vi "TaskCreationEvents.vi"(8 "error in (no error)":errorcluster, 11 "DAQmx(AI) in":refnum<class "DAQmx(AI).lvclass">) -> (0 "error out":errorcluster, 3 "DAQmx(AI) out":refnum<class "DAQmx(AI).lvclass">)   [LabVIEW 2019, in "DAQmx(AI).lvclass"]
uses:
  DAQmx(AI).lvclass
  Typedefs/ScalingEvent--Cluster.ctl
  Typedefs/Scaling(MapRange)--Cluster.ctl
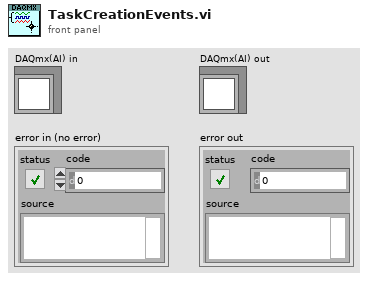
[diagram p1: front panel]
types:
  T1 = typedef "DAQmx(AI).lvclass/ScalingEvent--Cluster.ctl" = cluster{"Scale Name":string, "Units":string, "Range":T2}
  T2 = typedef "DAQmx(AI).lvclass/Scaling(MapRange)--Cluster.ctl" = cluster{"Minimum":dbl, "Maximum":dbl}
  T3 = typedef "DAQmx(AI).lvclass/PublicEvents--Cluster.ctl" = cluster{"Value Changed":refnum<user-event>, "Task Configuration":refnum<user-event>, "Scaling":refnum<user-event>}
  T4 = typedef "DAQmx(AI).lvclass/Configuration--Cluster.ctl" = cluster{"PhysChan":tag, "Period (ms)":i64, "input terminal cfg":i32, "minimum value":dbl, "maximum value":dbl, "units":T5, "task name":string, "TDMS File Path":path, "Group Name":string}
  T5 = typedef "DAQmx(AI).lvclass/Units -- Enum.ctl" = enum16{"Volts", "Amps", "Deg F", "Deg C", "Deg R", "Kelvins", "Strain", "Ohms", "Hz", "Seconds", "Meters", "Inches", "Degrees", "Radians", "Ticks", "g", "m/s^2", "m/s", "in/s", "Pascals", "Newtons", "Pounds", "kgf", "psi", "bar", "Nm", "oz-in", "lb-in", "lb-ft", "Volts/Volt", "mVolts/Volt", "From TEDS"}
  T6 = typedef "DAQmx(AI).lvclass/Scaling--Cluster.ctl" = cluster{"Scale Name":string, "Scale Type":T7, "Scaled Units":string, "Linear":T8, "Map Range":T2, "Polynomial":T9, "Table":T10}
  T7 = typedef "DAQmx(AI).lvclass/ScalingType--Enum.ctl" = enum16{"No scaling", "Linear", "Map Range", "Polynomial", "Table"}
  T8 = typedef "DAQmx(AI).lvclass/Scaling(Linear)--Cluster.ctl" = cluster{"Slope":dbl, "Intercept":dbl}
  T9 = typedef "DAQmx(AI).lvclass/Scaling(Polynomial)--Cluster.ctl" = cluster{"forward coeff":dbl[], "reverse coeff":dbl[]}
  T10 = typedef "DAQmx(AI).lvclass/Scaling(Table)--Cluster.ctl" = cluster{"scaled values":dbl[], "pres-scaled values":dbl[]}
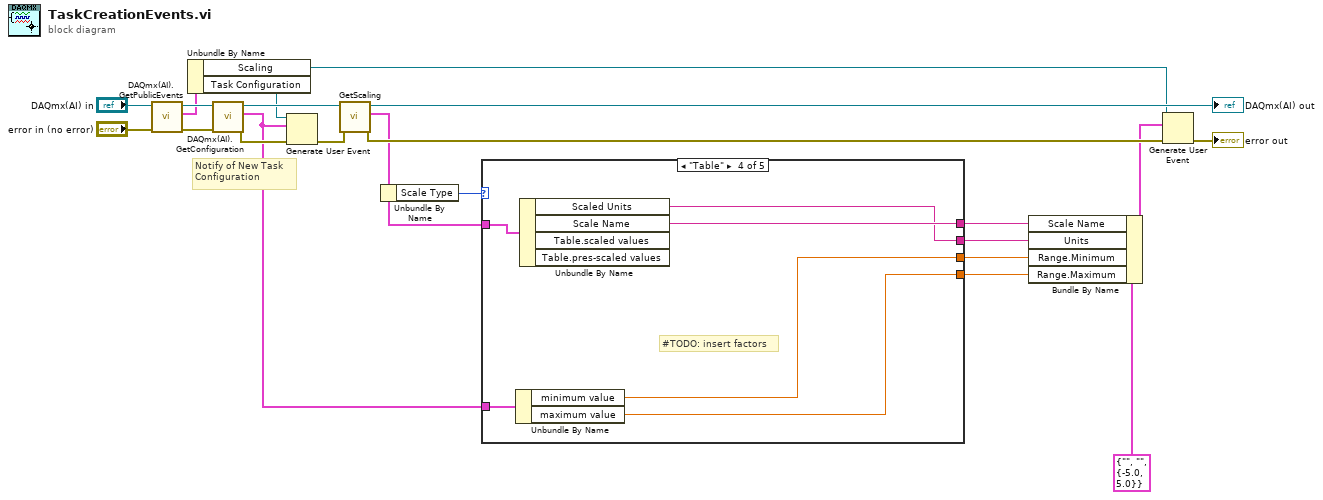
[diagram p0: block diagram]
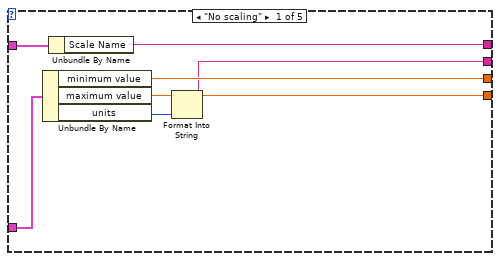
[diagram p2: hidden frame]
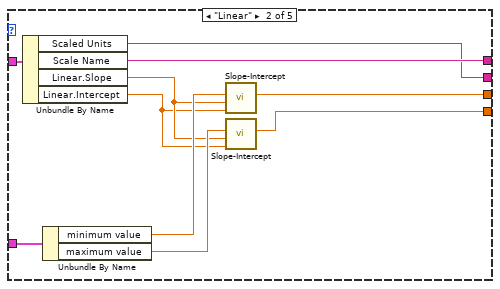
[diagram p3: hidden frame]
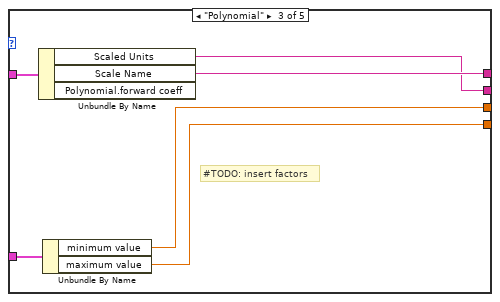
[diagram p4: hidden frame]
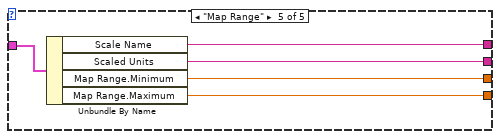
[diagram p5: hidden frame]
diagram:
  # "Notify of New Task\nConfiguration"
  n1 = call "DAQmx(AI).GetPublicEvents.vi"("error in (no error)"="error in (no error)", "Subsystem"="DAQmx(AI) in") -> ("error out"=w15:errorcluster, "DAQmx(AI) Public Events"=w11:T3, "Subsystem out"=w14:refnum<class "DAQmx(AI).lvclass">)  [unwired: 7 in]
  n2 = Unbundle By Name(w11) -> ("Scaling"=w18:refnum<user-event>, "Task Configuration"=w10:refnum<user-event>)
  n3 = call "DAQmx(AI).GetConfiguration.vi"("error in (no error)"=w15, "Subsystem"=w14) -> ("error out"=w16:errorcluster, "Configuration"=w4:T4, "Subsystem out"=w19:refnum<class "DAQmx(AI).lvclass">)  [unwired: 7 in]
  n4 = Generate User Event(user event=w10, event data cluster=w4, error in=w16) -> (error out=w22:errorcluster)  [unwired: 1 in, 1 out]
  n5 = call "GetScaling.vi"("error in (no error)"=w22, "Subsystem"=w19) -> ("error out"=w21:errorcluster, "Scaling"=w5:T6, "Subsystem out"=→"DAQmx(AI) out":refnum<class "DAQmx(AI).lvclass">)  [unwired: 6 in, 1 out]
  n6 = Unbundle By Name(w5) -> ("Scale Type"=w6:T7)
  n7 = case shown="\"Table\"" w6 {
    tunnel: [w29 w39 w45 w51 w52] -> w8
    tunnel: w5 -> [w28 w38 w44 w50 w56]
    tunnel: w4 -> [w27 w37 w43 w49 _]
    tunnel: [w26 w34 w40 w46 w55] -> w3
    tunnel: [w24 w36 w42 w48 w53] -> w2
    tunnel: [w23 w30 w41 w47 w54] -> w1
    frame "No scaling" {
      n8 = Unbundle By Name(w27) -> ("minimum value"=w26:dbl, "maximum value"=w23:dbl, "units"=w25:T5)
      n9 = Unbundle By Name(w28) -> ("Scale Name"=w29:string)
      n10 = Format Into String(w25) -> (resulting string=w24:string)  [unwired: 3 in, 1 out]
    }
    frame "Linear" {
      n11 = Unbundle By Name(w38) -> ("Scaled Units"=w36:string, "Scale Name"=w39:string, "Linear.Slope"=w32:dbl, "Linear.Intercept"=w31:dbl)
      n12 = Unbundle By Name(w37) -> ("minimum value"=w35:dbl, "maximum value"=w33:dbl)
      n13 = call "Slope-Intercept.vi"("Intercept"=w31, "Slope"=w32, "Value"=w35) -> ("Scaled Value"=w34:dbl)  [unwired: 8 in]
      n14 = call "Slope-Intercept.vi"("Intercept"=w31, "Slope"=w32, "Value"=w33) -> ("Scaled Value"=w30:dbl)  [unwired: 8 in]
    }
    frame "Polynomial" {
      # "#TODO: insert factors"
      n15 = Unbundle By Name(w44) -> ("Scaled Units"=w42:string, "Scale Name"=w45:string)  [unwired: 1 out]
      n16 = Unbundle By Name(w43) -> ("minimum value"=w40:dbl, "maximum value"=w41:dbl)
    }
    frame "Table" {
      # "#TODO: insert factors"
      n17 = Unbundle By Name(w49) -> ("minimum value"=w46:dbl, "maximum value"=w47:dbl)
      n18 = Unbundle By Name(w50) -> ("Scaled Units"=w48:string, "Scale Name"=w51:string)  [unwired: 2 out]
    }
    frame "Map Range" {
      n19 = Unbundle By Name(w56) -> ("Scale Name"=w52:string, "Scaled Units"=w53:string, "Map Range.Minimum"=w55:dbl, "Map Range.Maximum"=w54:dbl)
    }
  }
  n20 = Bundle By Name(cluster=T1 {"Scale Name"="", "Units"="", "Range"={"Minimum"=-5.0, "Maximum"=5.0}} ("Scaling Event"), "Scale Name"=w8, "Units"=w2, "Range.Minimum"=w3, "Range.Maximum"=w1) -> (w7:T1)
  n21 = Generate User Event(user event=w18, event data cluster=w7, error in=w21) -> (error out=→"error out":errorcluster)  [unwired: 1 in, 1 out]
